vi "SISTEMA NUMERICO.vi"() -> ()   [LabVIEW 2013]
panel:
  out "Parte decimale":dbl
  out "Parte intera":dbl
  in  "stop":bool
  out "ERRORE":bool
  out "RISULTATO":dbl format="%#.8g"
  in  "BASE":dbl
  in  "C-3":dbl
  in  "C-2":dbl
  in  "C-1":dbl
  in  "C2":dbl
  in  "C1":dbl
  in  "C0":dbl
  in  "C3":dbl
  # ","
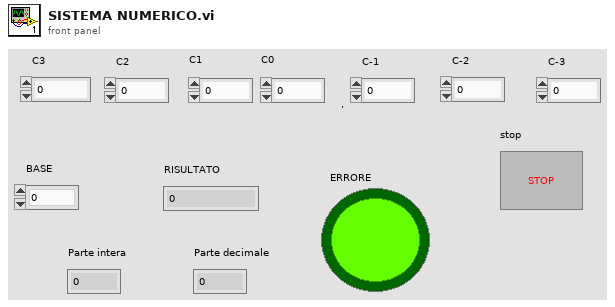
[diagram p1: front panel]
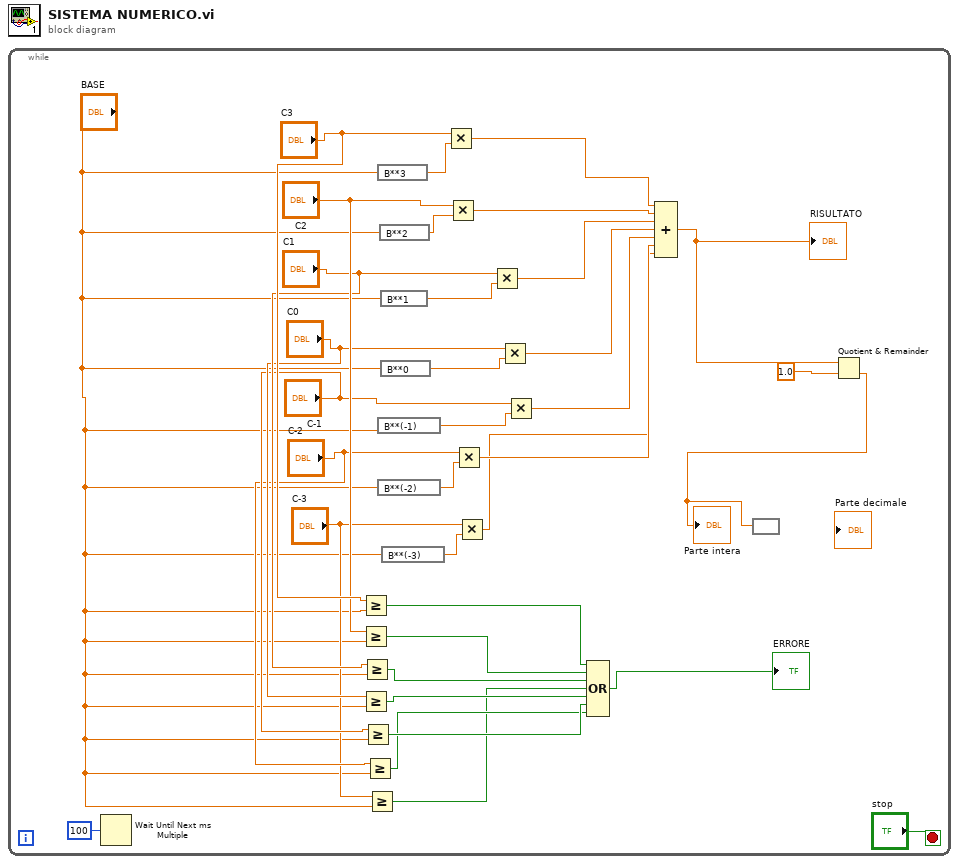
[diagram p0: block diagram]
diagram:
  n1 = while {
    stop <- "stop" stop-if-true
    n2 = Wait Until Next ms Multiple(millisecond multiple=u32 100) -> ()  [unwired: 1 out]
    n3 = Greater Or Equal?(x="C3", y="BASE") -> (x >= y?=w13:bool)
    n4 = Greater Or Equal?(x="C2", y="BASE") -> (x >= y?=w12:bool)
    n5 = Greater Or Equal?(x="C0", y="BASE") -> (x >= y?=w10:bool)
    n6 = Greater Or Equal?(x="C1", y="BASE") -> (x >= y?=w11:bool)
    n7 = Greater Or Equal?(x="C-1", y="BASE") -> (x >= y?=w9:bool)
    n8 = Greater Or Equal?(x="C-2", y="BASE") -> (x >= y?=w8:bool)
    n9 = Greater Or Equal?(x="C-3", y="BASE") -> (x >= y?=w6:bool)
    n10 = expression code="B**3"("BASE") -> (w35:dbl)
    n11 = expression code="B**(-1)"("BASE") -> (w32:dbl)
    n12 = expression code="B**(-2)"("BASE") -> (w25:dbl)
    n13 = expression code="B**2"("BASE") -> (w30:dbl)
    n14 = expression code="B**1"("BASE") -> (w34:dbl)
    n15 = expression code="B**0"("BASE") -> (w33:dbl)
    n16 = expression code="B**(-3)"("BASE") -> (w24:dbl)
    n17 = Multiply(x="C3", y=w35) -> (x*y=w31:dbl)
    n18 = Multiply(x="C2", y=w30) -> (x*y=w29:dbl)
    n19 = Multiply(x="C-2", y=w25) -> (x*y=w23:dbl)
    n20 = Multiply(x="C-3", y=w24) -> (x*y=w22:dbl)
    n21 = Multiply(x="C1", y=w34) -> (x*y=w28:dbl)
    n22 = Multiply(x="C0", y=w33) -> (x*y=w27:dbl)
    n23 = Multiply(x="C-1", y=w32) -> (x*y=w26:dbl)
    n24 = Compound Arithmetic op=OR(w13, w12, w11, w6, w10, w9, w8) -> (→"ERRORE":bool)
    n25 = Compound Arithmetic op=ADD(w31, w29, w28, w27, w26, w23, w22) -> (w3:dbl)
    "RISULTATO" <- w3
    n26 = Quotient & Remainder(x=w3, y=1.0) -> (floor(x/y)=w1:dbl)  [unwired: 1 out]
    "Parte intera" <- w1
    n27 = expression code=""(w1) -> ()  [unwired: 1 out]
  }
